vi "ActivateMenu.vi"(7 "Menu.lvclass":refnum<class "Menu.lvclass">, 8 "error in (no error)":errorcluster caption="错误输入（无错误）", 9 "MenuClassArray":refnum<class "Menu.lvclass">[](array[class]), 11 "listbox 输入":refnum<class "listbox.lvclass">) -> (0 "error out":errorcluster caption="错误输出", 3 "listbox 输出":refnum<class "listbox.lvclass">)   [LabVIEW 2016, in "listbox.lvclass"]
uses:
  listbox.lvclass
  LNK/Parent Class/Menu.lvclass
  listbox.lvclass/listbox.ctl
  LNK/Parent Class/Menu.lvclass/Menu.ctl
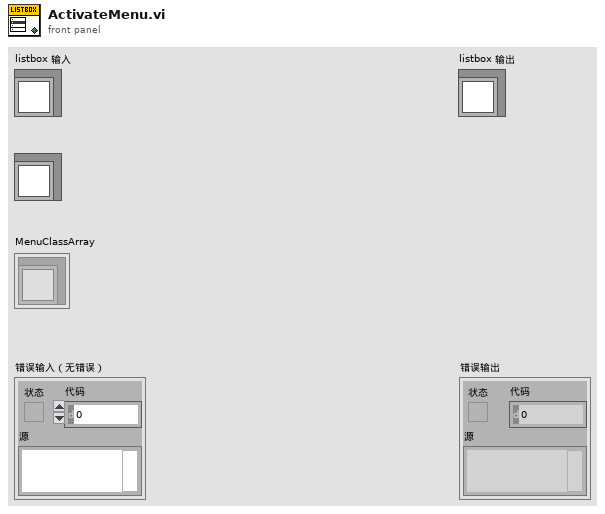
[diagram p1: front panel]
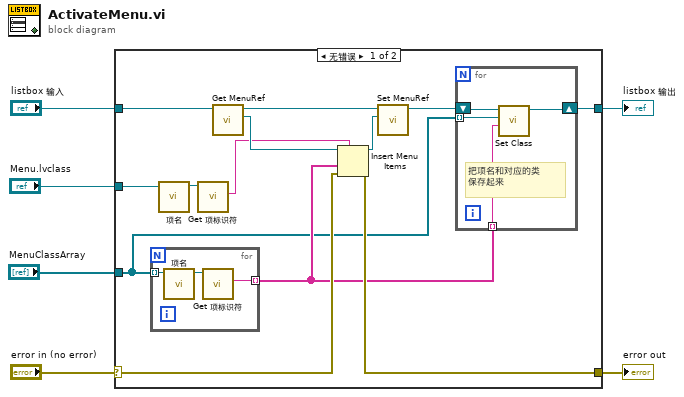
[diagram p0: block diagram]
diagram:
  n1 = case shown="无错误" "error in (no error)" {
    selector: "error in (no error)" -> [w12 w28]
    tunnel: [w11 w28] -> w5
    tunnel: [w9 w27] -> w3
    tunnel: "listbox 输入" -> [w19 w27]
    tunnel: "Menu.lvclass" -> [w15 _]
    tunnel: "MenuClassArray" -> [w7 _]
    frame No Error {
      n2 = for {
        tunnel: w7 -> [w26] mode=indexing
        tunnel: [w24] -> w8 mode=indexing
        n3 = call-dynamic "项名.vi"("LNK 输入"=w26) -> ("LNK 输出"=w25:refnum<class "Menu.lvclass">)  [unwired: 9 in, 1 out]
        n4 = call "Get 项标识符.vi"("LNK in"=w25) -> ("项标识符"=w24:string)  [unwired: 9 in, 1 out]
      }
      n5 = call-dynamic "项名.vi"("LNK 输入"=w15) -> ("LNK 输出"=w16:refnum<class "Menu.lvclass">)  [unwired: 9 in, 1 out]
      n6 = call "Get 项标识符.vi"("LNK in"=w16) -> ("项标识符"=w14:string)  [unwired: 9 in, 1 out]
      n7 = call "Get MenuRef.vi"("listbox in"=w19) -> ("MenuRef"=w17:refnum<k9>, "listbox out"=w18:refnum<class "listbox.lvclass">)  [unwired: 9 in]
      n8 = Insert Menu Items(5:w14, 6:w12, 7:w8, 9:w17) -> (0:w11:errorcluster, 3:w13:refnum<k9>)  [unwired: 2 in, 1 out]
      n9 = call "Set MenuRef.vi"("MenuRef"=w13, "listbox in"=w18) -> ("listbox out"=w10:refnum<class "listbox.lvclass">)  [unwired: 9 in]
      n10 = for {
        shift-right: [w22] -> w9
        shift-left: w10 -> [w23]
        tunnel: w8 -> [w21] mode=indexing
        tunnel: w7 -> [w20] mode=indexing
        # "把项名和对应的类\n保存起来"
        n11 = call "Set Class.vi"("项标识符"=w21, "LNK.lvclass"=w20, "listbox 输入"=w23) -> ("listbox 输出"=w22:refnum<class "listbox.lvclass">)  [unwired: 7 in, 1 out]
      }
    }
    frame Error {
    }
  }
  "error out" <- w5
  "listbox 输出" <- w3
